vi "Read Write Settings.vi"(0 "Settings In":T1={"Save Options"={"Primary Storage Location"=path "", "Backup Storage Location"=path "", "Enable Primary"=FALSE, "Enable Secondary"=FALSE, "Save Image as"=enum."RAW"}, "Other Settings"={"Show Image Averaging Option"=TRUE, "Component Name Prefix"=""}, "PLC Parameters"={"Initialize Parameters"={"VISA  Port"="", "Baud Rate"=0}, "Wakeup Bit (Set)"={"Address"=0, "Set/Reset"=FALSE}, "Incoming Bit (Get)"={"Address"=0, "Set/Reset"=FALSE}, "Acknowledge Bit (Set)"={"Address"=0, "Set/Reset"=FALSE}}}, 11 "error in (no error)":errorcluster, 13 "Operations":enum16{"Read Settings", "Write Settings"}(ring)=enum."Write Settings") -> (4 "Settings Out":T1={"Save Options"={"Primary Storage Location"=path "", "Backup Storage Location"=path "", "Enable Primary"=FALSE, "Enable Secondary"=FALSE, "Save Image as"=enum."RAW"}, "Other Settings"={"Show Image Averaging Option"=TRUE, "Component Name Prefix"=""}, "PLC Parameters"={"Initialize Parameters"={"VISA  Port"="", "Baud Rate"=0}, "Wakeup Bit (Set)"={"Address"=0, "Set/Reset"=FALSE}, "Incoming Bit (Get)"={"Address"=0, "Set/Reset"=FALSE}, "Acknowledge Bit (Set)"={"Address"=0, "Set/Reset"=FALSE}}}, 15 "error out":errorcluster)   [LabVIEW 2022 SP3]
uses:
  Controls/Application Settings.ctl
  <vilib>/Utility/config.llb/Read Key (Boolean).vi
  <vilib>/Utility/config.llb/Read Key (U32).vi
  <vilib>/Utility/config.llb/Read Key (Path).vi
  <vilib>/Utility/config.llb/Read Key (String).vi
  <vilib>/Utility/config.llb/Write Key (Boolean).vi
  <vilib>/Utility/config.llb/Write Key (U32).vi
  <vilib>/Utility/config.llb/Write Key (Path).vi
  <vilib>/Utility/config.llb/Write Key (String).vi
  <vilib>/Utility/config.llb/NI_LVConfig.lvlib
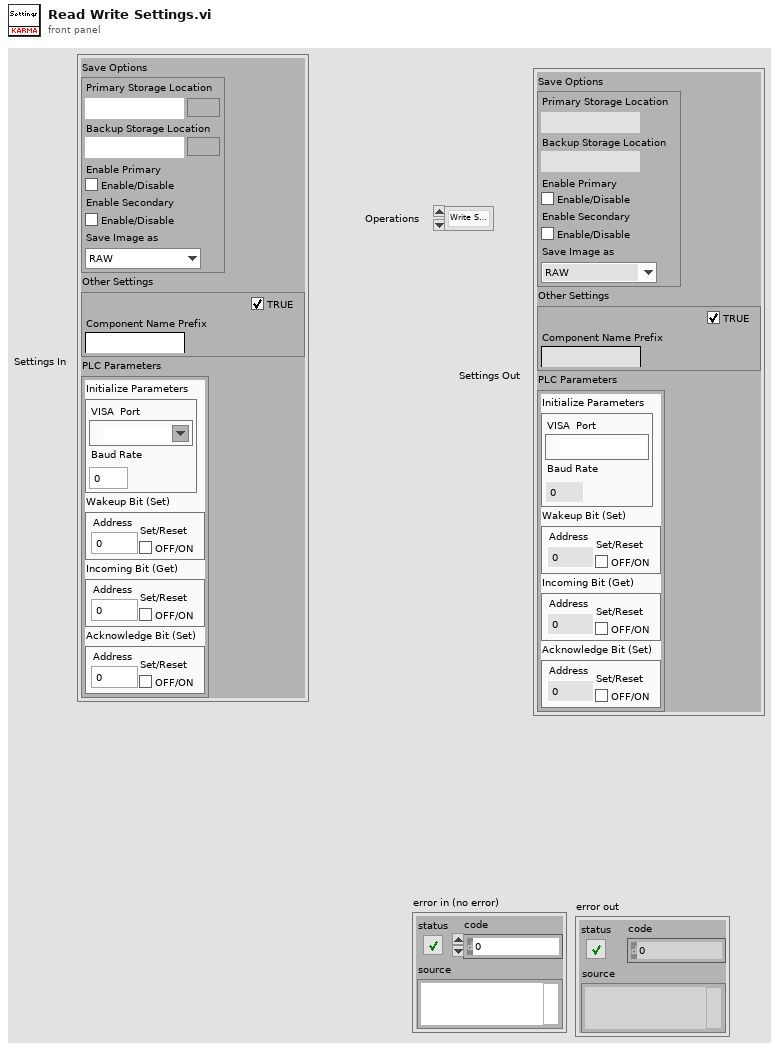
[diagram p1: front panel]
types:
  T1 = typedef "Application Settings.ctl" = cluster{"Save Options":cluster{"Primary Storage Location":path, "Backup Storage Location":path, "Enable Primary":bool, "Enable Secondary":bool, "Save Image as":enum16{"RAW", "TIFF"}}, "Other Settings":cluster{"Show Image Averaging Option":bool, "Component Name Prefix":string}, "PLC Parameters":cluster{"Initialize Parameters":cluster{"VISA  Port":refnum<visa-resource-name>, "Baud Rate":u32}, "Wakeup Bit (Set)":cluster{"Address":u16, "Set/Reset":bool}, "Incoming Bit (Get)":cluster{"Address":u16, "Set/Reset":bool}, "Acknowledge Bit (Set)":cluster{"Address":u16, "Set/Reset":bool}}}
  T2 = typedef "Paths.ctl" = cluster{"Configuration":path, "Event Logs":path, "Error Logs":path, "Configuration.ini":path}
  T3 = typedef "NI_LVConfig.lvlib/Config Data RefNum.ctl" = refnum<k1>
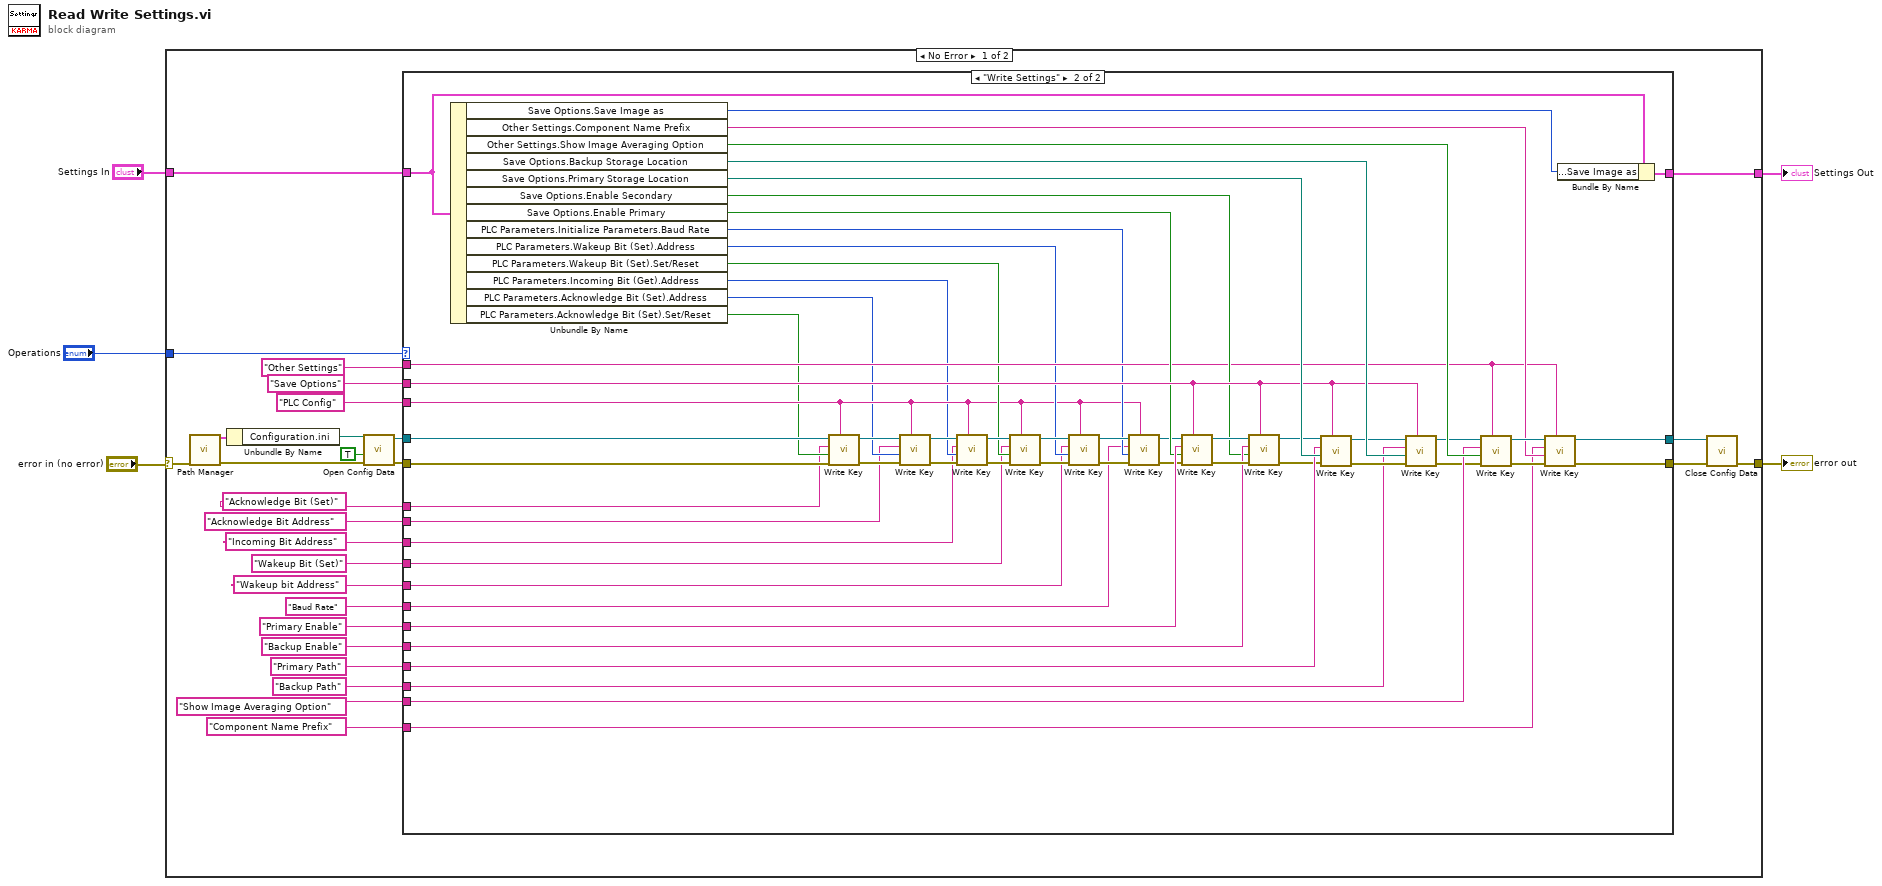
[diagram p0: block diagram]
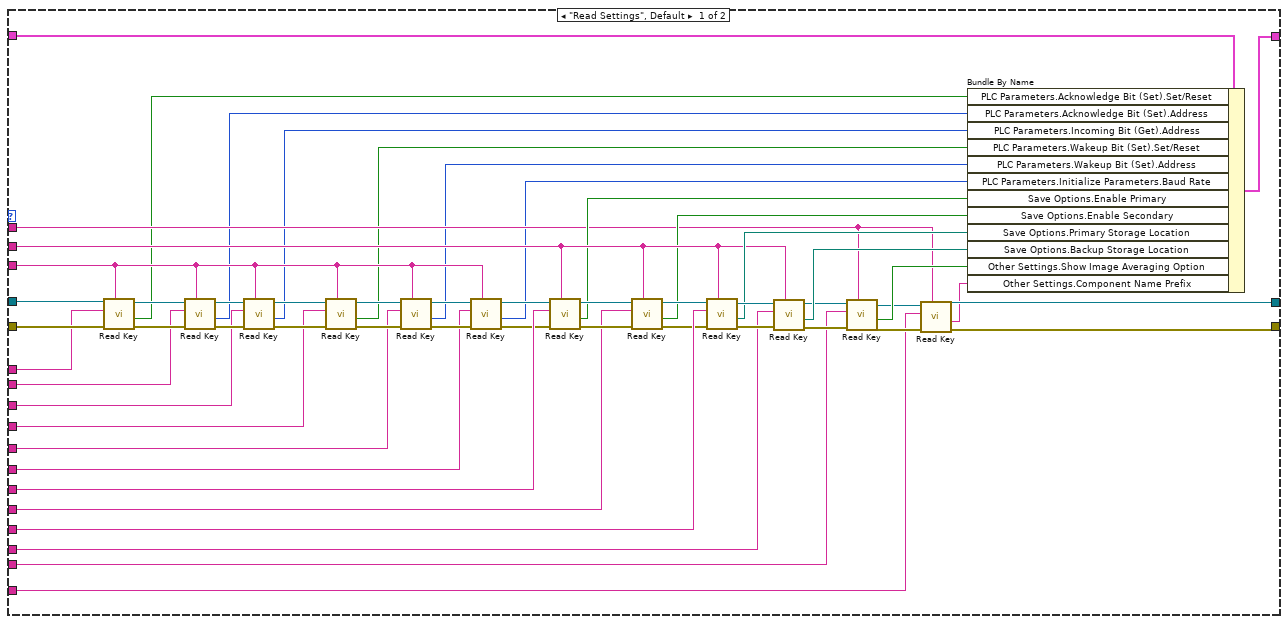
[diagram p2: hidden frame]
diagram:
  n1 = case shown="No Error" "error in (no error)" {
    selector: "error in (no error)" -> [w33 w145]
    tunnel: [w32 w145] -> w4
    tunnel: "Operations" -> [w31 _]
    tunnel: "Settings In" -> [w30 _]
    tunnel: [w29 _] -> w1
    frame No Error {
      n2 = call "Path Manager.vi"("error in (no error)"=w33) -> ("Cluster"=w28:T2, "Error out"=w27:errorcluster)  [unwired: 13 in]
      n3 = Unbundle By Name(w28) -> ("Configuration.ini"=w24:path)
      n4 = call <vilib>:"Open Config Data.vi"("error in (no error)"=w27, "create file if necessary (T)"=TRUE, "configuration file path"=w24) -> ("error out"=w26:errorcluster, "refnum"=w23:T3)  [unwired: 6 in, 1 out]
      n5 = case shown="\"Write Settings\"" w31 {
        tunnel: [w65 w122] -> w25
        tunnel: w30 -> [w84 w90]
        tunnel: w26 -> [w60 w103]
        tunnel: w23 -> [w53 w118]
        tunnel: [w64 w123] -> w22
        tunnel: "Backup Path" ("key") -> [w85 w140]
        tunnel: "Primary Path" ("key") -> [w86 w139]
        tunnel: "Save Options" ("section") -> [w79 w134]
        tunnel: "PLC Config" ("section") -> [w46 w107]
        tunnel: [w81 w91] -> w29
        tunnel: "Primary Enable" ("key") -> [w74 w133]
        tunnel: "Backup Enable" ("key") -> [w75 w132]
        tunnel: "Show Image Averaging Option" ("key") -> [w69 w128]
        tunnel: "Other Settings" ("section") -> [w63 w120]
        tunnel: "Component Name Prefix" ("key") -> [w62 w119]
        tunnel: "Baud Rate" ("key") -> [w40 w97]
        tunnel: "Wakeup bit Address" ("key") -> [w38 w96]
        tunnel: "Wakeup Bit (Set)" ("key") -> [w43 w95]
        tunnel: "Incoming Bit Address" ("key") -> [w42 w94]
        tunnel: "Acknowledge Bit Address" ("key") -> [w44 w93]
        tunnel: "Acknowledge Bit (Set)" ("key") -> [w45 w92]
        frame "Read Settings", Default {
          n6 = call-poly <vilib>:"Read Key.vi"("section"=w46, "error in (no error)"=w60, "key"=w45, "refnum"=w53) -> ("error out"=w59:errorcluster, "value"=w34:bool, "refnum out"=w52:T3)  [unwired: 4 in, 1 out]
          n7 = call-poly <vilib>:"Read Key.vi"("section"=w46, "error in (no error)"=w59, "key"=w44, "refnum"=w52) -> ("error out"=w58:errorcluster, "value"=w35:u32, "refnum out"=w51:T3)  [unwired: 4 in, 1 out]
          n8 = call-poly <vilib>:"Read Key.vi"("section"=w46, "error in (no error)"=w58, "key"=w42, "refnum"=w51) -> ("error out"=w57:errorcluster, "value"=w36:u32, "refnum out"=w50:T3)  [unwired: 4 in, 1 out]
          n9 = call-poly <vilib>:"Read Key.vi"("section"=w46, "error in (no error)"=w57, "key"=w43, "refnum"=w50) -> ("error out"=w56:errorcluster, "value"=w37:bool, "refnum out"=w49:T3)  [unwired: 4 in, 1 out]
          n10 = call-poly <vilib>:"Read Key.vi"("section"=w46, "error in (no error)"=w56, "key"=w38, "refnum"=w49) -> ("error out"=w55:errorcluster, "value"=w39:u32, "refnum out"=w48:T3)  [unwired: 4 in, 1 out]
          n11 = call-poly <vilib>:"Read Key.vi"("section"=w46, "error in (no error)"=w55, "key"=w40, "refnum"=w48) -> ("error out"=w54:errorcluster, "value"=w41:u32, "refnum out"=w47:T3)  [unwired: 4 in, 1 out]
          n12 = call-poly <vilib>:"Read Key.vi"("section"=w79, "error in (no error)"=w54, "key"=w74, "refnum"=w47) -> ("error out"=w80:errorcluster, "value"=w72:bool, "refnum out"=w78:T3)  [unwired: 4 in, 1 out]
          n13 = call-poly <vilib>:"Read Key.vi"("section"=w79, "error in (no error)"=w80, "key"=w75, "refnum"=w78) -> ("error out"=w76:errorcluster, "value"=w73:bool, "refnum out"=w77:T3)  [unwired: 4 in, 1 out]
          n14 = call-poly <vilib>:"Read Key.vi"("section"=w79, "error in (no error)"=w76, "key"=w86, "refnum"=w77) -> ("error out"=w88:errorcluster, "value"=w83:path, "refnum out"=w87:T3)  [unwired: 4 in, 1 out]
          n15 = call-poly <vilib>:"Read Key.vi"("section"=w79, "error in (no error)"=w88, "key"=w85, "refnum"=w87) -> ("error out"=w70:errorcluster, "value"=w82:path, "refnum out"=w71:T3)  [unwired: 4 in, 1 out]
          n16 = call-poly <vilib>:"Read Key.vi"("section"=w63, "error in (no error)"=w70, "key"=w69, "refnum"=w71) -> ("error out"=w66:errorcluster, "value"=w68:bool, "refnum out"=w67:T3)  [unwired: 4 in, 1 out]
          n17 = call-poly <vilib>:"Read Key.vi"("section"=w63, "error in (no error)"=w66, "key"=w62, "refnum"=w67) -> ("error out"=w65:errorcluster, "value"=w61:string, "refnum out"=w64:T3)  [unwired: 4 in, 1 out]
          n18 = Bundle By Name(cluster=w84, "PLC Parameters.Acknowledge Bit (Set).Set/Reset"=w34, "PLC Parameters.Acknowledge Bit (Set).Address"=w35, "PLC Parameters.Incoming Bit (Get).Address"=w36, "PLC Parameters.Wakeup Bit (Set).Set/Reset"=w37, "PLC Parameters.Wakeup Bit (Set).Address"=w39, "PLC Parameters.Initialize Parameters.Baud Rate"=w41, "Save Options.Enable Primary"=w72, "Save Options.Enable Secondary"=w73, "Save Options.Primary Storage Location"=w83, "Save Options.Backup Storage Location"=w82, "Other Settings.Show Image Averaging Option"=w68, "Other Settings.Component Name Prefix"=w61) -> (w81:T1)
        }
        frame "Write Settings" {
          n19 = Unbundle By Name(w90) -> ("Save Options.Save Image as"=w89:enum16{"RAW", "TIFF"}, "Other Settings.Component Name Prefix"=w121:string, "Other Settings.Show Image Averaging Option"=w129:bool, "Save Options.Backup Storage Location"=w142:path, "Save Options.Primary Storage Location"=w143:path, "Save Options.Enable Secondary"=w130:bool, "Save Options.Enable Primary"=w131:bool, "PLC Parameters.Initialize Parameters.Baud Rate"=w110:u32, "PLC Parameters.Wakeup Bit (Set).Address"=w109:u16, "PLC Parameters.Wakeup Bit (Set).Set/Reset"=w108:bool, "PLC Parameters.Incoming Bit (Get).Address"=w104:u16, "PLC Parameters.Acknowledge Bit (Set).Address"=w105:u16, "PLC Parameters.Acknowledge Bit (Set).Set/Reset"=w106:bool)
          n20 = call-poly <vilib>:"Write Key.vi"("section"=w107, "error in (no error)"=w103, "value"=w106, "key"=w92, "refnum"=w118) -> ("error out"=w102:errorcluster, "refnum out"=w117:T3)  [unwired: 4 in, 1 out]
          n21 = call-poly <vilib>:"Write Key.vi"("section"=w107, "error in (no error)"=w102, "value"=w105, "key"=w93, "refnum"=w117) -> ("error out"=w101:errorcluster, "refnum out"=w116:T3)  [unwired: 4 in, 1 out]
          n22 = call-poly <vilib>:"Write Key.vi"("section"=w107, "error in (no error)"=w101, "value"=w104, "key"=w94, "refnum"=w116) -> ("error out"=w100:errorcluster, "refnum out"=w115:T3)  [unwired: 4 in, 1 out]
          n23 = call-poly <vilib>:"Write Key.vi"("section"=w107, "error in (no error)"=w100, "value"=w108, "key"=w95, "refnum"=w115) -> ("error out"=w99:errorcluster, "refnum out"=w114:T3)  [unwired: 4 in, 1 out]
          n24 = call-poly <vilib>:"Write Key.vi"("section"=w107, "error in (no error)"=w99, "value"=w109, "key"=w96, "refnum"=w114) -> ("error out"=w98:errorcluster, "refnum out"=w113:T3)  [unwired: 4 in, 1 out]
          n25 = call-poly <vilib>:"Write Key.vi"("section"=w107, "error in (no error)"=w98, "value"=w110, "key"=w97, "refnum"=w113) -> ("error out"=w112:errorcluster, "refnum out"=w111:T3)  [unwired: 4 in, 1 out]
          n26 = call-poly <vilib>:"Write Key.vi"("section"=w134, "error in (no error)"=w112, "value"=w131, "key"=w133, "refnum"=w111) -> ("error out"=w137:errorcluster, "refnum out"=w138:T3)  [unwired: 4 in, 1 out]
          n27 = call-poly <vilib>:"Write Key.vi"("section"=w134, "error in (no error)"=w137, "value"=w130, "key"=w132, "refnum"=w138) -> ("error out"=w135:errorcluster, "refnum out"=w136:T3)  [unwired: 4 in, 1 out]
          n28 = call-poly <vilib>:"Write Key.vi"("section"=w134, "error in (no error)"=w135, "value"=w143, "key"=w139, "refnum"=w136) -> ("error out"=w144:errorcluster, "refnum out"=w141:T3)  [unwired: 4 in, 1 out]
          n29 = call-poly <vilib>:"Write Key.vi"("section"=w134, "error in (no error)"=w144, "value"=w142, "key"=w140, "refnum"=w141) -> ("error out"=w126:errorcluster, "refnum out"=w127:T3)  [unwired: 4 in, 1 out]
          n30 = call-poly <vilib>:"Write Key.vi"("section"=w120, "error in (no error)"=w126, "value"=w129, "key"=w128, "refnum"=w127) -> ("error out"=w124:errorcluster, "refnum out"=w125:T3)  [unwired: 4 in, 1 out]
          n31 = call-poly <vilib>:"Write Key.vi"("section"=w120, "error in (no error)"=w124, "value"=w121, "key"=w119, "refnum"=w125) -> ("error out"=w122:errorcluster, "refnum out"=w123:T3)  [unwired: 4 in, 1 out]
          n32 = Bundle By Name(cluster=w90, "Save Options.Save Image as"=w89) -> (w91:T1)
        }
      }
      n33 = call <vilib>:"Close Config Data.vi"("error in (no error)"=w25, "refnum"=w22) -> ("error out"=w32:errorcluster)  [unwired: 8 in, 1 out]
    }
    frame Error {
    }
  }
  "error out" <- w4
  "Settings Out" <- w1
